vi "Write Interface Name.vi"(8 "error in (no error)":errorcluster, 10 "Interface Name":T1(ring), 11 "DeviceNET in":refnum<class "DeviceNET.lvclass">) -> (0 "error out":errorcluster, 3 "DeviceNET out":refnum<class "DeviceNET.lvclass">)   [LabVIEW 2016, in "DeviceNET.lvclass"]
uses:
  DeviceNET.lvclass
  DeviceNET.lvclass/DeviceNET.ctl
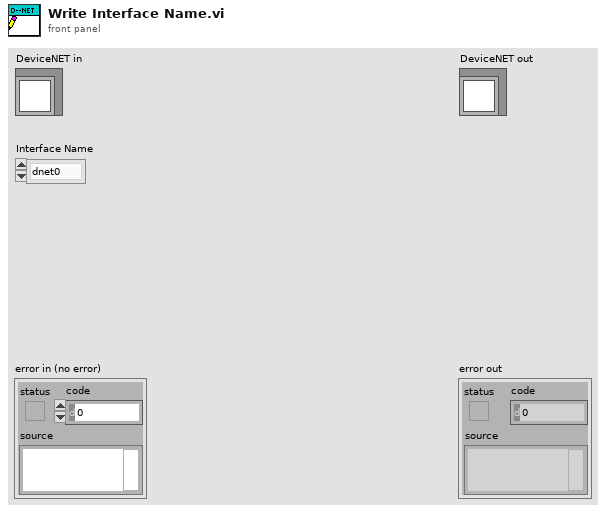
[diagram p1: front panel]
types:
  T1 = enum16{"dnet0", "dnet1", "dnet2", "dnet3", "dnet4", "dnet5", "dnet6", "dnet7", "dnet8", "dnet9", "dnet10", "dnet11", "dnet12", "dnet13", "dnet14", "dnet15", "dnet16", "dnet17", "dnet18", "dnet19", "dnet20", "dnet21", "dnet22", "dnet23", "dnet24", "dnet25", "dnet26", "dnet27", "dnet28", "dnet29", "dnet30", "dnet31"}
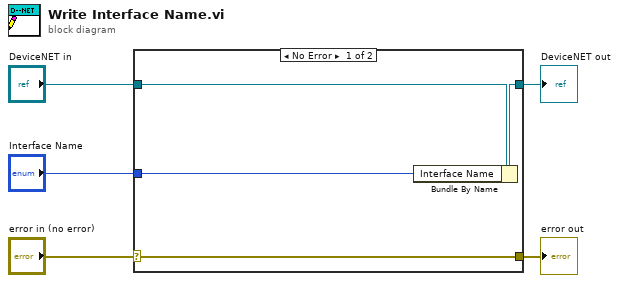
[diagram p0: block diagram]
diagram:
  n1 = case shown="No Error" "error in (no error)" {
    selector: "error in (no error)" -> [w9 w10]
    tunnel: [w9 w10] -> w4
    tunnel: [w7 w11] -> w2
    tunnel: "DeviceNET in" -> [w8 w11]
    tunnel: "Interface Name" -> [w6 _]
    frame No Error {
      n2 = Bundle By Name(cluster=w8, "Interface Name"=w6) -> (w7:refnum<class "DeviceNET.lvclass">)
    }
    frame Error {
    }
  }
  "error out" <- w4
  "DeviceNET out" <- w2
